vi "Igniter.vi"(0 "Ignition":bool) -> (3 "Solenoids":bool[](array[boolean]), 6 "Spark Plug":bool)   [LabVIEW 2016]
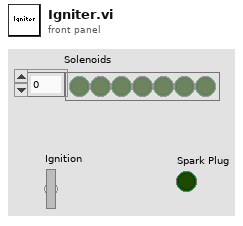
[diagram p1: front panel]
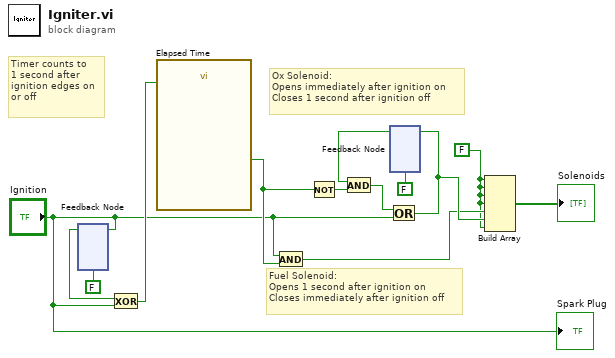
[diagram p0: block diagram]
diagram:
  w2 = FALSE
  # "Timer counts to\n1 second after\nignition edges on\nor off"
  # "Ox Solenoid:\nOpens immediately after ignition on\nCloses 1 second after ignition off"
  # "Fuel Solenoid:\nOpens 1 second after ignition on\nCloses immediately after ignition off"
  n1 = feedback #1(FALSE) -> (w9:bool)
  n2 = feedback-in #1("Ignition") -> ()
  n3 = Exclusive Or(1:"Ignition", 2:w9) -> (0:w7:bool)
  n4 = call "Elapsed Time"("Reset"=w7) -> ("Time has Elapsed"=w8:bool)  [unwired: 11 in, 7 out]
  n5 = And(x="Ignition", y=w8) -> (x .and. y?=w3:bool)
  n6 = Not(x=w8) -> (.not. x?=w12:bool)
  n7 = feedback #2(FALSE) -> (w13:bool)
  n8 = And(x=w13, y=w12) -> (x .and. y?=w6:bool)
  n9 = Or(x=w6, y="Ignition") -> (x .or. y?=w4:bool)
  n10 = feedback-in #2(w4) -> ()
  n11 = Build Array(w2, w2, w2, w2, w3, w4, w2) -> (→"Solenoids":bool[])
  "Spark Plug" <- "Ignition"
